vi "Begin.vi"(8 "error in (no error)":errorcluster, 9 "Reverse Solenoid Channel":T1, 10 "Forward Solenoid Channel":T1, 11 "SingleSolenoid in":refnum<class "SingleSolenoid.lvclass">) -> (0 "error out":errorcluster, 3 "SingleSolenoid out":refnum<class "SingleSolenoid.lvclass">)   [LabVIEW 2018, in "Pneumatics control.lvlib" / "SingleSolenoid.lvclass"]
uses:
  SingleSolenoid.lvclass
  <vilib>/Rock Robotics/WPI/Solenoid/WPI_SolenoidChannel.ctl
  Solenoids.lvclass
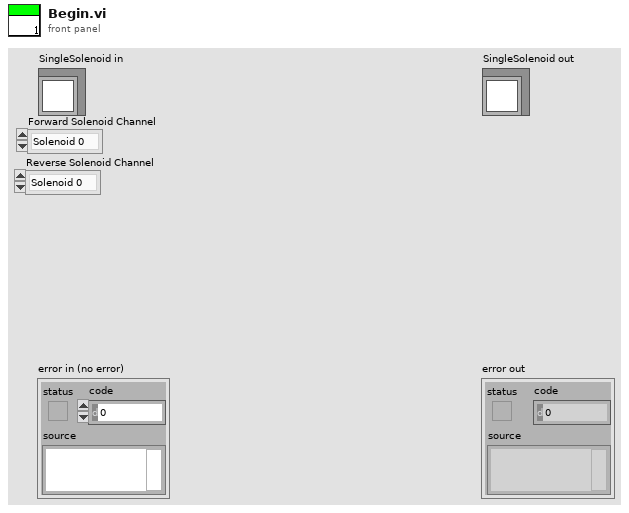
[diagram p1: front panel]
types:
  T1 = typedef "WPI_SolenoidChannel.ctl" = enum8{"Solenoid 0", "Solenoid 1", "Solenoid 2", "Solenoid 3", "Solenoid 4", "Solenoid 5", "Solenoid 6", "Solenoid 7", "Invalid"}
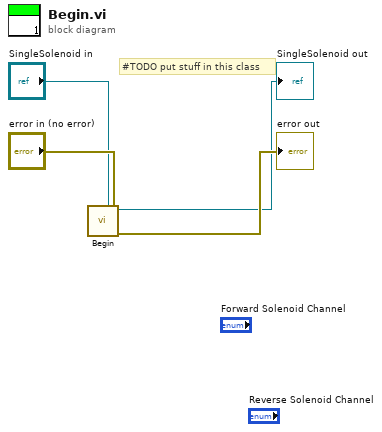
[diagram p0: block diagram]
diagram:
  # "#TODO put stuff in this class"
  n1 = call-parent "Begin.vi"("error in (no error)"="error in (no error)", "Solenoids in"="SingleSolenoid in") -> ("error out"=→"error out":errorcluster, "Solenoids out"=→"SingleSolenoid out":refnum<class "SingleSolenoid.lvclass">)  [unwired: 8 in]
